vi "Keyence.Main-Scan.Product.vi"(7 "Slot":T4, 8 "error in":errorcluster, 10 "Code in":T1, 11 "Code sets in":T5={"Ready"=FALSE, "DoubleOrder"=FALSE, "OrderDone"=FALSE, "AllowSingleSlot"=FALSE, "TunedA"=FALSE, "TunedB"=FALSE, "CheckDM"=FALSE, "ThresholdA"=0, "ThresholdB"=0, "Plate"=enum."Wabco", "ImgPath"=path "", "Variant"={"State"=enum."Init", "ImgPath"=path "", "WabcoPlate"="", "WabcoProduct"="", "ClientProduct"="", "ClientPlate"="", "TotalQuantity"=0, "OrderQuantity"=0, "Serial"=0, "Wabco"={"LaserJob"="", "AdditionalTxt"="037", "FactoryCode"="", "RevID"=0, "ForkID"=0, "FailuresLimit"=0, "GlobalCnt"=0, "Bank"=0, "SerialFormat"=enum."6 dig", "CoordA"={"X"=0.0, "Y"=0.0, "Angle"=0.0}, "CoordB"={"X"=0.0, "Y"=0.0, "Angle"=0.0}, "DMCconfig"=0}, "Client"={"LaserJob"="", "AdditionalTxt"="", "FactoryCode"="037", "RevID"=0, "ForkID"=0, "FailuresLimit"=0, "GlobalCnt"=0, "Bank"=0, "SerialFormat"=enum."6 dig", "CoordA"={"X"=0.0, "Y"=0.0, "Angle"=0.0}, "CoordB"={"X"=0.0, "Y"=0.0, "Angle"=0.0}, "DMCconfig"=0}}}) -> (0 "error out":errorcluster, 2 "Code out":T1)   [LabVIEW 2016]
uses:
  Sequence/Sequence.Code.Sets.ctl
  Sequence/Sequence.PlateType.ctl
  Logger/Logger.Variant.Sets.ctl
  Station/Station.Changeover.State.vi
  Station/Station.Plate.Properties.ctl
  Sequence/Sequence.Code.SerialFormat.ctl
  V7310/LowLevel/V7310.Job.Sets.ctl
  Station/Station.ProductSlot.ctl
  Sequence/Sequence.Prod.StatusData.ctl
  Sequence/Sequence.Step.Status.ctl
  Sequence/Sequence.Test.BreakReason.ctl
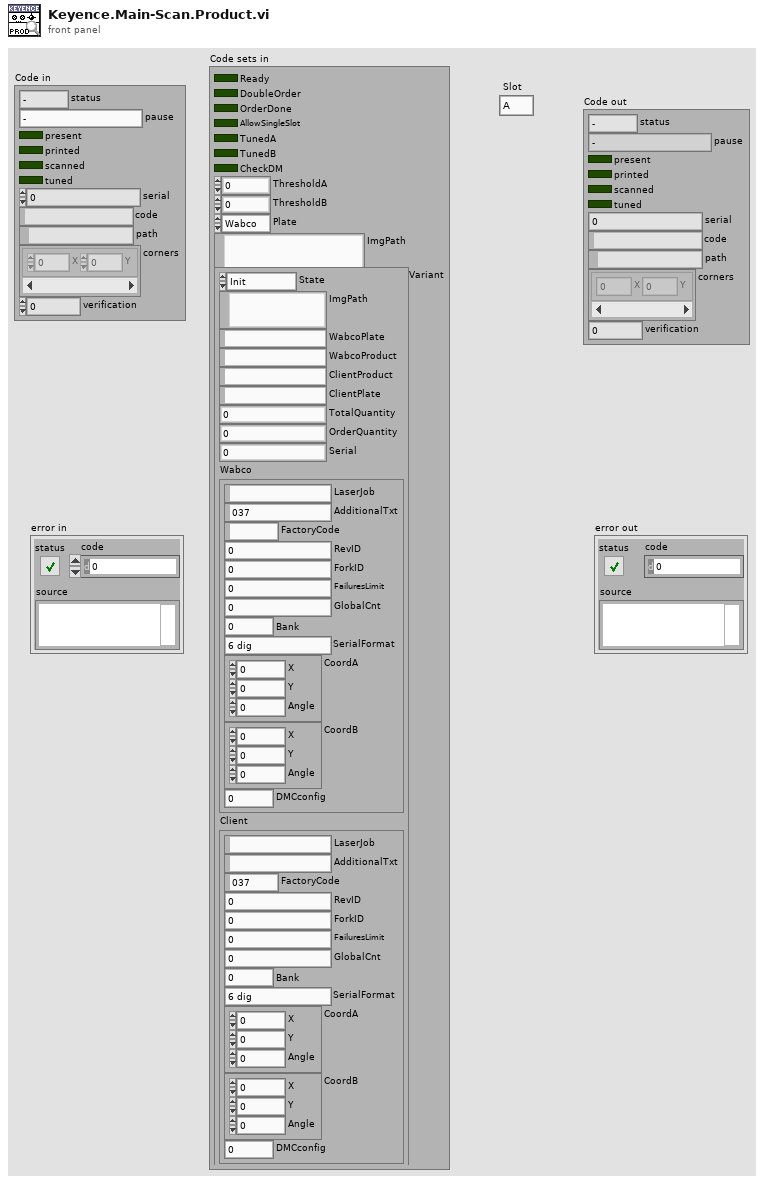
[diagram p1: front panel]
types:
  T1 = typedef "Sequence.Prod.StatusData.ctl" = cluster{"status":T2, "pause":T3, "present":bool, "printed":bool, "scanned":bool, "tuned":bool, "serial":i32, "code":string, "path":path, "corners":cluster{"X":i32, "Y":i32}[], "verification":u8}
  T2 = typedef "Sequence.Step.Status.ctl" = enum16{"-", "Pending", "Running", "Skipped", "Passed", "Failed", "Done", "Error", "Aborted", "Stopped"}
  T3 = typedef "Sequence.Test.BreakReason.ctl" = enum16{"-", "NOK container", "OK container", "Rev empty", "Rev missing", "Rev wrong", "Fork missing", "Fork wrong", "NOK limit", "Unload failure", "Single slot", "Part done", "Err: Prod move work", "Err: Prod move home", "Err: Prod lift work", "Err: Prod lift home", "Err: Prod Arm Work", "Err: Prod Arm NOK", "Err: Prod Arm OK", "Err: Prod NOK suck", "Err: Prod NOK drop", "Err: Prod OK missing", "Err: Prod OK suck", "Err: Prod OK drop"}
  T4 = typedef "Station.ProductSlot.ctl" = enum8{"A", "B"}
  T5 = typedef "Sequence.Code.Sets.ctl" = cluster{"Ready":bool, "DoubleOrder":bool, "OrderDone":bool, "AllowSingleSlot":bool, "TunedA":bool, "TunedB":bool, "CheckDM":bool, "ThresholdA":u8, "ThresholdB":u8, "Plate":T6, "ImgPath":path, "Variant":T7}
  T6 = typedef "Sequence.PlateType.ctl" = enum16{"Wabco", "Client"}
  T7 = typedef "Logger.Variant.Sets.ctl" = cluster{"State":T8, "ImgPath":path, "WabcoPlate":string, "WabcoProduct":string, "ClientProduct":string, "ClientPlate":string, "TotalQuantity":u16, "OrderQuantity":u16, "Serial":i32, "Wabco":T9, "Client":T9}
  T8 = typedef "Station.Changeover.State.vi" = enum16{"Init", "Scaning", "NOK", "Wait for ack", "Ready"}
  T9 = typedef "Station.Plate.Properties.ctl" = cluster{"LaserJob":string, "AdditionalTxt":string, "FactoryCode":string, "RevID":u8, "ForkID":u8, "FailuresLimit":u16, "GlobalCnt":i32, "Bank":u8, "SerialFormat":T10, "CoordA":T11, "CoordB":T11, "DMCconfig":i32}
  T10 = typedef "Sequence.Code.SerialFormat.ctl" = enum8{"", "6 dig", "7 dig"}
  T11 = typedef "V7310.Job.Sets.ctl" = cluster{"X":dbl, "Y":dbl, "Angle":dbl}
  T12 = typedef "Keyence.CodeDetails.ctl" = cluster{"text":string, "status":bool, "corners":cluster{"X":i32, "Y":i32}[], "level":u8, "class":string, "path":path}
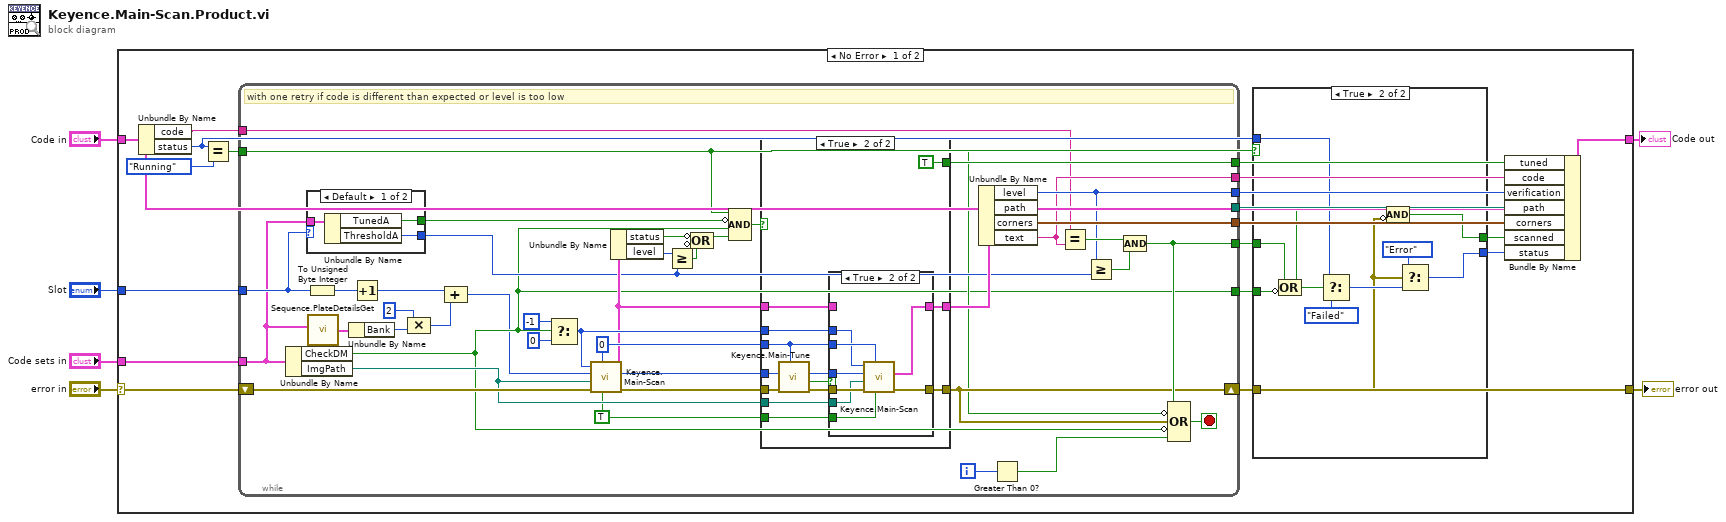
[diagram p0: block diagram]
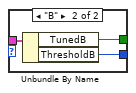
[diagram p5: hidden frame]
diagram:
  n1 = case shown="No Error" "error in" {
    selector: "error in" -> [w25 w109]
    tunnel: [w19 w109] -> w5
    tunnel: "Code sets in" -> [w20 _]
    tunnel: "Slot" -> [w22 _]
    tunnel: "Code in" -> [w11 w108]
    tunnel: [w21 w108] -> w1
    frame No Error {
      n2 = Unbundle By Name(w11) -> ("code"=w12:string, "status"=w8:T2)
      n3 = Equal?(x=w8, y=Sequence.Step.Status."Running") -> (x = y?=w9:bool)
      n4 = while {
        tunnel: [w73] -> w24
        tunnel: [w72] -> w23
        tunnel: w22 -> [w70]
        tunnel: w20 -> [w42]
        tunnel: [w51] -> w18
        tunnel: [w49] -> w17
        tunnel: [w44] -> w16
        tunnel: [w52] -> w15
        shift-right: [w46] -> w19
        shift-left: w25 -> [w77]
        tunnel: [w48] -> w7
        tunnel: w12 -> [w43]
        tunnel: w9 -> [w45]
        i -> [w54]
        stop <- w53 stop-if-true
        w65 = TRUE ("get img (F)")
        w64 = 0 ("Idx")
        # "with one retry if code is different than expected or level is too low"
        n5 = Unbundle By Name(w42) -> ("CheckDM"=w44:bool, "ImgPath"=w76:path)
        n6 = case shown="Default" w70 {
          tunnel: w42 -> [w104 w107]
          tunnel: [w103 w106] -> w60
          tunnel: [w102 w105] -> w58
          frame Default {
            n7 = Unbundle By Name(w104) -> ("TunedA"=w103:bool, "ThresholdA"=w102:u8)
          }
          frame "B" {
            n8 = Unbundle By Name(w107) -> ("TunedB"=w106:bool, "ThresholdB"=w105:u8)
          }
        }
        n9 = To Unsigned Byte Integer(number=w70) -> (unsigned 8bit integer=w75:u8)
        n10 = call "Sequence.PlateDetailsGet.vi"("Code in"=w42) -> ("PlateDetails"=w41:T9)  [unwired: 9 in, 1 out]
        n11 = Unbundle By Name(w41) -> ("Bank"=w39:u8)
        n12 = Increment(x=w75) -> (x+1=w74:u8)
        n13 = Compound Arithmetic op=MULTIPLY(u8 2 ("value"), w39) -> (w37:u8)
        n14 = Compound Arithmetic op=ADD(w74, w37) -> (w40:u8)
        n15 = Select(t=-1 ("Retries"), s=w44, f=0 ("Retries")) -> (s? t:f=w62:i32)
        n16 = call "Keyence.Main-Scan.vi"("get img (F)"=w65, "Idx"=w64, "error in"=w77, "imgpath"=w76, "Bank"=w40, "Retries (-1: Default)"=w62) -> ("error out"=w63:errorcluster, "Code"=w61:T12)  [unwired: 3 in, 1 out]
        n17 = Unbundle By Name(w61) -> ("status"=w67:bool, "level"=w59:u8)
        n18 = Greater Or Equal?(x=w59, y=w58) -> (x >= y?=w56:bool)
        n19 = Compound Arithmetic op=OR(invert w67, invert w56) -> (w57:bool)
        n20 = Compound Arithmetic op=AND(w45, invert w60, w44, w57) -> (w66:bool)
        n21 = case shown="True" w66 {
          tunnel: w65 -> [_ w91]
          tunnel: w64 -> [_ w89]
          tunnel: w63 -> [w79 w90]
          tunnel: [w79 w87] -> w46
          tunnel: w40 -> [_ w86]
          tunnel: w62 -> [_ w85]
          tunnel: w76 -> [_ w84]
          tunnel: w61 -> [w78 w83]
          tunnel: [w78 w82] -> w71
          tunnel: [_ TRUE ("Tuned")] -> w51
          frame False {
          }
          frame True {
            n22 = call "Keyence.Main-Tune.vi"("Idx"=w89, "error in"=w90, "Bank"=w86) -> ("error out"=w88:errorcluster, "Tuned"=w81:bool)  [unwired: 5 in, 2 out]
            n23 = case shown="True" w81 {
              tunnel: w91 -> [_ w101]
              tunnel: w89 -> [_ w100]
              tunnel: w88 -> [w93 w99]
              tunnel: [w93 w98] -> w87
              tunnel: w86 -> [_ w97]
              tunnel: w85 -> [_ w96]
              tunnel: w84 -> [_ w95]
              tunnel: w83 -> [w92 _]
              tunnel: [w92 w94] -> w82
              frame False {
              }
              frame True {
                n24 = call "Keyence.Main-Scan.vi"("get img (F)"=w101, "Idx"=w100, "error in"=w99, "imgpath"=w95, "Bank"=w97, "Retries (-1: Default)"=w96) -> ("error out"=w98:errorcluster, "Code"=w94:T12)  [unwired: 3 in, 1 out]
              }
            }
          }
        }
        n25 = Unbundle By Name(w71) -> ("level"=w49:u8, "path"=w72:path, "corners"=w73:cluster{"X":i32, "Y":i32}[], "text"=w48:string)
        n26 = Greater Than 0?(x=w54) -> (x > 0?=w47:bool)
        n27 = Equal?(x=w43, y=w48) -> (x = y?=w50:bool)
        n28 = Greater Or Equal?(x=w49, y=w58) -> (x >= y?=w55:bool)
        n29 = Compound Arithmetic op=AND(w50, w55) -> (w52:bool)
        n30 = Compound Arithmetic op=OR(w52, invert w45, w46, invert w44, w47) -> (w53:bool)
      }
      n31 = case shown="True" w9 {
        tunnel: w19 -> [_ w29]
        tunnel: w16 -> [_ w35]
        tunnel: w15 -> [_ w34]
        tunnel: [_ w27] -> w14
        tunnel: [w26 w32] -> w13
        tunnel: w8 -> [w26 w30]
        frame False {
        }
        frame True {
          n32 = Compound Arithmetic op=OR(w34, invert w35) -> (w28:bool)
          n33 = Select(t=w30, s=w28, f=Sequence.Step.Status."Failed" ("status")) -> (s? t:f=w31:T2)
          n34 = Compound Arithmetic op=AND(w28, invert w29) -> (w27:bool)
          n35 = Select(t=Sequence.Step.Status."Error" ("status"), s=w29, f=w31) -> (s? t:f=w32:T2)
        }
      }
      n36 = Bundle By Name(cluster=w11, "tuned"=w18, "code"=w7, "verification"=w17, "path"=w23, "corners"=w24, "scanned"=w14, "status"=w13) -> (w21:T1)
    }
    frame Error {
    }
  }
  "error out" <- w5
  "Code out" <- w1
